vi "WordTableRead.vi"() -> ()   [LabVIEW 2012]
panel:
  in  "Column":i32=4
  in  "Row":i32=4
  in  "Word._Application":refnum<k7>
  out "Read Cell":string
  out "error out":errorcluster
  in  "template (empty)":path
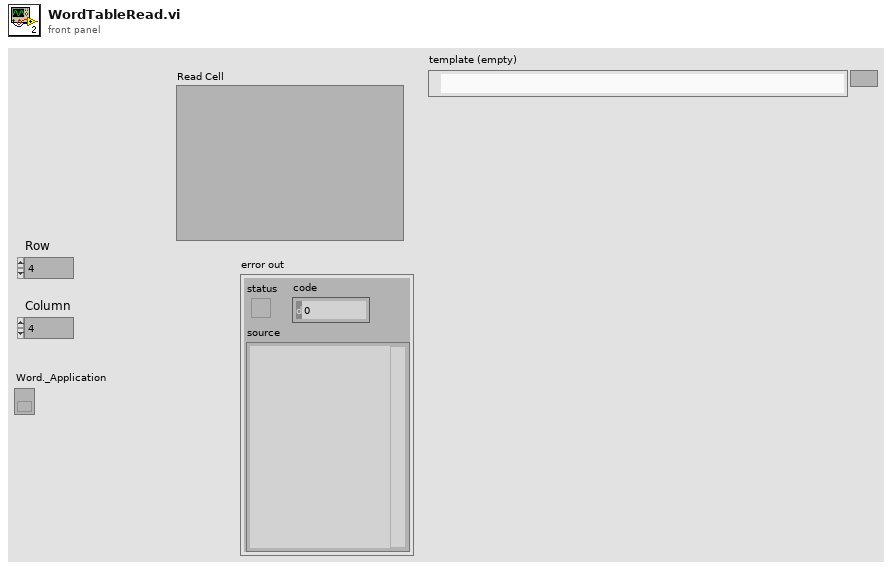
[diagram p1: front panel]
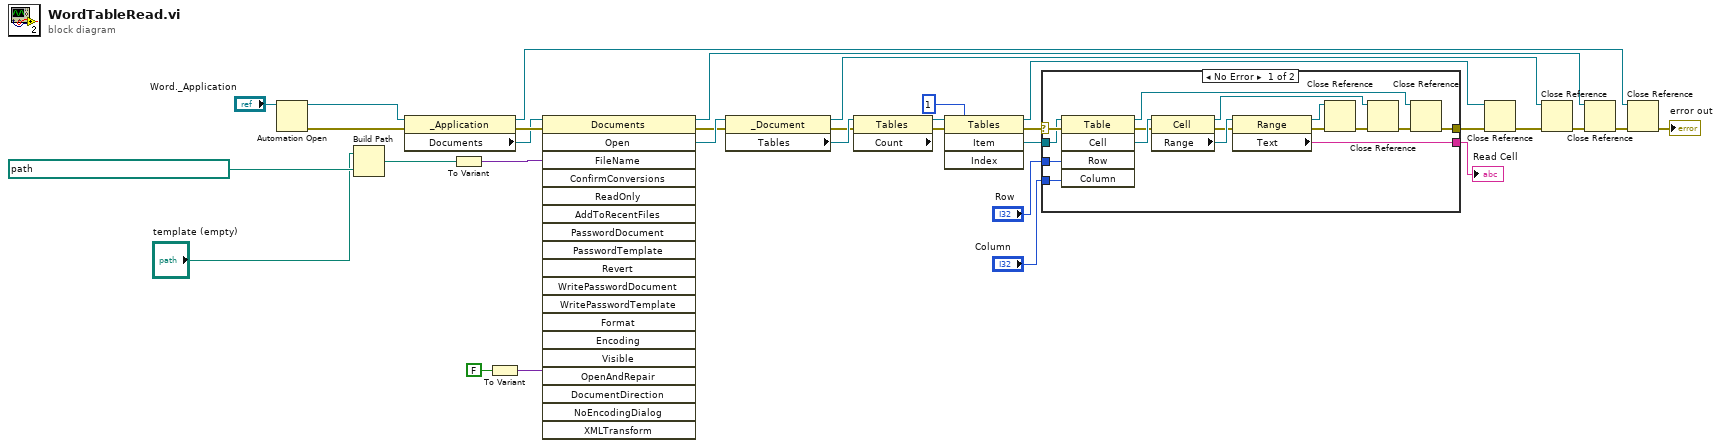
[diagram p0: block diagram]
diagram:
  n1 = Automation Open(Automation Refnum="Word._Application") -> (Automation Refnum=w13:refnum<k7>, error out=w26:errorcluster)  [unwired: 3 in]
  n2 = Build Path(base path="template (empty)", name or relative path=path "PP-E-04-06H MT、AT生產確認單.doc") -> (appended path=w2:path)
  n3 = property class="_Application"(reference=w13, error in=w26) -> (reference out=w14:refnum<k7>, error out=w30:errorcluster, "Documents"=w28:refnum<k7>)
  n4 = To Variant(anything=w2) -> (Variant=w27:variant)
  n5 = To Variant(anything=FALSE) -> (Variant=w5:variant)
  n6 = invoke class="Documents" method="Open"(reference=w28, error in=w30, "FileName"=w27, "Visible"=w5) -> (reference out=w7:refnum<k7>, error out=w23:errorcluster, "Open"=w25:refnum<k7>)  [unwired: 15 in, 16 out]
  n7 = property class="_Document"(reference=w25, error in=w23) -> (reference out=w15:refnum<k7>, error out=w17:errorcluster, "Tables"=w20:refnum<k7>)
  n8 = property class="Tables" props=["Count"](reference=w20, error in=w17) -> (reference out=w19:refnum<k7>, error out=w18:errorcluster)  [unwired: 1 out]
  n9 = invoke class="Tables" method="Item"(reference=w19, error in=w18, "Index"=1) -> (reference out=w16:refnum<k7>, error out=w22:errorcluster, "Item"=w24:refnum<k7>)  [unwired: 1 in, 1 out]
  n10 = case shown="No Error" w22 {
    selector: w22 -> [w42 w49]
    tunnel: "Row" -> [w46 _]
    tunnel: "Column" -> [w45 _]
    tunnel: [w34 w49] -> w12
    tunnel: [w38 _] -> w29
    tunnel: w24 -> [w37 _]
    frame No Error {
      n11 = invoke class="Table" method="Cell"(reference=w37, error in=w42, "Row"=w46, "Column"=w45) -> (reference out=w36:refnum<k7>, error out=w41:errorcluster, "Cell"=w48:refnum<k7>)  [unwired: 1 in, 2 out]
      n12 = property class="Cell"(reference=w48, error in=w41) -> (reference out=w44:refnum<k7>, error out=w40:errorcluster, "Range"=w47:refnum<k7>)
      n13 = property class="Range"(reference=w47, error in=w40) -> (reference out=w33:refnum<k7>, error out=w39:errorcluster, "Text"=w38:string)
      n14 = Close Reference(reference=w33, error in (no error)=w39) -> (error out=w43:errorcluster)
      n15 = Close Reference(reference=w44, error in (no error)=w43) -> (error out=w35:errorcluster)
      n16 = Close Reference(reference=w36, error in (no error)=w35) -> (error out=w34:errorcluster)
    }
    frame Error {
    }
  }
  "Read Cell" <- w29
  n17 = Close Reference(reference=w16, error in (no error)=w12) -> (error out=w11:errorcluster)
  n18 = Close Reference(reference=w15, error in (no error)=w11) -> (error out=w6:errorcluster)
  n19 = Close Reference(reference=w7, error in (no error)=w6) -> (error out=w10:errorcluster)
  n20 = Close Reference(reference=w14, error in (no error)=w10) -> (error out=→"error out":errorcluster)
